vi "Stop Module.vi"(6 "Timeout to Wait for Stop (s) (-1: no timeout)":dbl=-1.0, 8 "error in":errorcluster, 9 "Wait for Module to Stop? (F)":bool, 10 "Origin":string) -> (0 "error out":errorcluster)   [LabVIEW 2024, in "IOLink.lvlib"]
doc: "Send the Stop request to the Module's Main.vi.\n\nIf <b>Wait for Module to Stop?</b> is TRUE, this VI will wait until the module main VI stops, and will timeout at the <b>Timeout to Wait for Stop</b> value. This value defaults to \"-1\", which means the VI will not timeout, and will always wait until the module main VI stops before completing execution.\n\nNote: The <b>Timeout to Wait for Stop</b> value is ignored if 'Wait for Module to Stop?' is set to FALSE.\n_____\nBased on DQMH Project Template 7.0.0.1280."
uses:
  IOLink.lvlib
  Stop Argument--cluster.ctl
  <vilib>/event_ctls.llb/usereventprio.ctl
panel:
  # "Note: The 'Timeout to Wait for Stop' value is ignored if 'Wait for Module to Stop?' is set to FALSE."
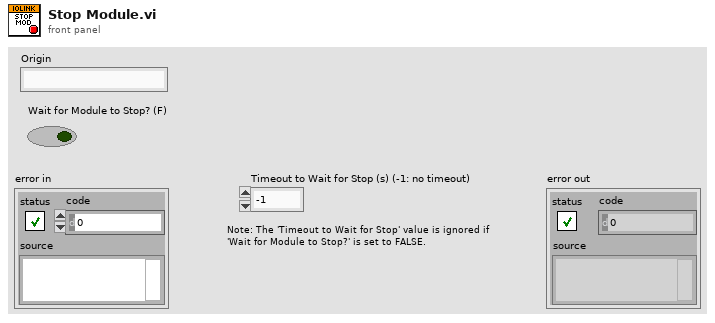
[diagram p1: front panel]
types:
  T1 = typedef "IOLink.lvlib/Stop Argument--cluster.ctl" = cluster{"Origin":string, "Exit via Stop Module Req?":bool, "Wait for Module to stop?":bool}
  T2 = typedef "usereventprio.ctl" = enum32{"high priority", "normal priority"}
  T3 = typedef "IOLink.lvlib/Request Events--cluster.ctl" = cluster{"Stop Module":refnum<user-event>, "Show Panel":refnum<user-event>, "Hide Panel":refnum<user-event>, "Get Module Execution Status":refnum<user-event>, "Show Diagram":refnum<user-event>}
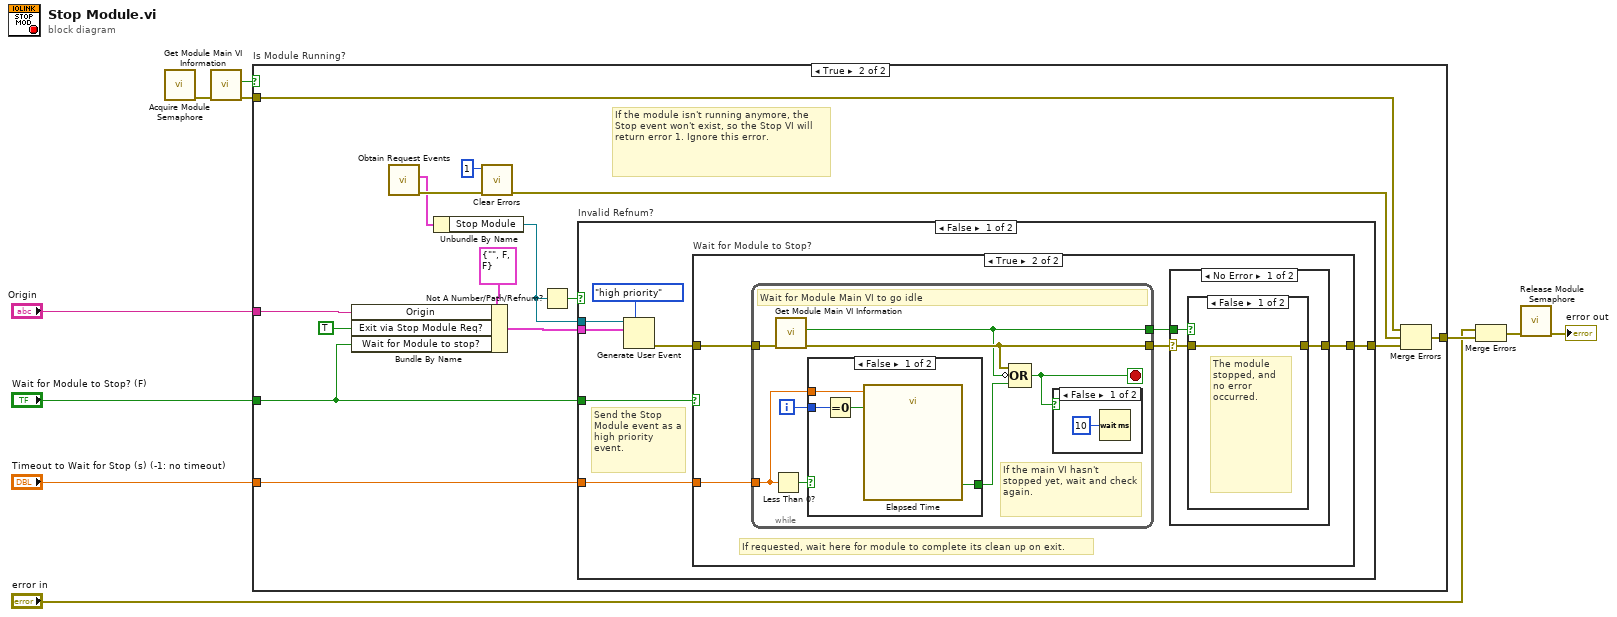
[diagram p0: block diagram]
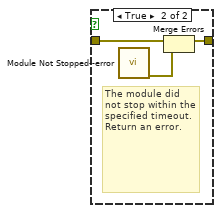
[diagram p4: hidden frame]
diagram:
  n1 = call "Acquire Module Semaphore.vi"() -> ("error out"=w4:errorcluster)  [unwired: 11 in]
  n2 = call "Get Module Main VI Information.vi"("error in"=w4) -> ("error out"=w7:errorcluster, "Is Module Running?"=w6:bool)  [unwired: 7 in, 2 out]
  n3 = case "Is Module Running?" shown="True" w6 {
    tunnel: [w11 w25] -> w10
    tunnel: "Origin" -> [_ w24]
    tunnel: w7 -> [w11 w16]
    tunnel: "Wait for Module to Stop? (F)" -> [_ w13]
    tunnel: "Timeout to Wait for Stop (s) (-1: no timeout)" -> [_ w12]
    frame False {
      # "The module is not running, there is no need to run the Stop Module code."
    }
    frame True {
      # "If the module isn't running anymore, the Stop event won't exist, so the Stop VI will return error 1. Ignore this error."
      n4 = Bundle By Name(cluster=T1 {"Origin"="", "Exit via Stop Module Req?"=FALSE, "Wait for Module to stop?"=FALSE} ("event data"), "Origin"=w24, "Exit via Stop Module Req?"=TRUE, "Wait for Module to stop?"=w13) -> (w19:T1)
      n5 = call "Obtain Request Events.vi"() -> ("error out"=w26:errorcluster, "IOLink Request Events"=w23:T3)  [unwired: 10 in]
      n6 = Unbundle By Name(w23) -> ("Stop Module"=w20:refnum<user-event>)
      n7 = call <vilib>:"Clear Errors.vi"("error in (no error)"=w26, "specific error code to clear (0: all)"=1) -> ("error out"=w15:errorcluster)  [unwired: 4 in, 1 out]
      n8 = Not A Number/Path/Refnum?(number/path/refnum=w20) -> (NaN/Path/Refnum?=w21:bool)
      n9 = case "Invalid Refnum?" shown="False" w21 {
        tunnel: [w28 _] -> w18
        tunnel: w20 -> [w33 _]
        tunnel: w19 -> [w31 _]
        tunnel: w13 -> [w29 _]
        tunnel: w12 -> [w27 _]
        frame False {
          # "Send the Stop Module event as a high priority event."
          n10 = Generate User Event(priority (normal)=usereventprio."high priority", user event=w33, event data cluster=w31) -> (error out=w30:errorcluster)  [unwired: 1 in, 1 out]
          n11 = case "Wait for Module to Stop?" shown="True" w29 {
            tunnel: w30 -> [w34 w38]
            tunnel: [w34 w36] -> w28
            tunnel: w27 -> [_ w39]
            frame False {
            }
            frame True {
              # "If requested, wait here for module to complete its clean up on exit."
              n12 = while {
                tunnel: w39 -> [w50]
                tunnel: w38 -> [w54]
                tunnel: [w53] -> w37
                tunnel: [w52] -> w35
                i -> [w55]
                stop <- w48 stop-if-true
                # "If the main VI hasn't stopped yet, wait and check again."
                # "Wait for Module Main VI to go idle"
                n13 = Less Than 0?(x=w50) -> (x < 0?=w49:bool)
                n14 = call "Get Module Main VI Information.vi"("error in"=w54) -> ("error out"=w53:errorcluster, "Is Module Running?"=w52:bool)  [unwired: 7 in, 2 out]
                n15 = case shown="False" w49 {
                  tunnel: w50 -> [w57 _]
                  tunnel: w55 -> [w59 _]
                  tunnel: [w58 _] -> w51
                  frame False {
                    n16 = Equal To 0?(x=w59) -> (x = 0?=w60:bool)
                    n17 = call "Elapsed Time"("Time Target (s)"=w57, "Reset"=w60) -> ("Time has Elapsed"=w58:bool)  [unwired: 10 in, 7 out]
                  }
                  frame True {
                    # "User specified a timeout of -1, so don't keep track of the elapsed time since this loop started."
                  }
                }
                n18 = Compound Arithmetic op=OR(w53, invert w52, w51) -> (w48:bool)
                n19 = case shown="False" w48 {
                  frame False {
                    n20 = Wait (ms)(milliseconds to wait=u32 10) -> ()  [unwired: 1 out]
                  }
                  frame True {
                  }
                }
              }
              n21 = case shown="No Error" w37 {
                selector: w37 -> [w41 w47]
                tunnel: [w40 w47] -> w36
                tunnel: w35 -> [w42 _]
                frame No Error {
                  n22 = case shown="False" w42 {
                    tunnel: w41 -> [w43 w46]
                    tunnel: [w43 w45] -> w40
                    frame False {
                      # "The module stopped, and no error occurred."
                    }
                    frame True {
                      # "The module did not stop within the specified timeout. Return an error."
                      n23 = call "Module Not Stopped--error.vi"() -> ("error out"=w44:errorcluster)  [unwired: 11 in]
                      n24 = Merge Errors(w46, w44) -> (w45:errorcluster)
                    }
                  }
                }
                frame Error {
                  # "An error occurred while waiting for the module to stop. Return that error."
                }
              }
            }
          }
        }
        frame True {
          # "Module is exiting. No need to send the standard \"not running\" error that is sent in other request VIs."
        }
      }
      n25 = Merge Errors(w16, w15, w18) -> (w25:errorcluster)
    }
  }
  n26 = Merge Errors("error in", w10) -> (w2:errorcluster)
  n27 = call "Release Module Semaphore.vi"("error in"=w2) -> ("error out"=→"error out":errorcluster)  [unwired: 10 in]
